vi "Obtain Broadcast Events.vi"(8 "error in (no error)":errorcluster, 10 "Create New?":bool) -> (0 "error out":errorcluster, 2 "Temperature-Module Broadcast Events":T1)   [LabVIEW 2021, in "Temperature-Module.lvlib"]
doc: "This VI Obtains/Creates the Broadcast events that will be used for other libraries to register to receive messages from the library that owns this VI.\n\n<b>NOTE</b>: The contents of this VI are automatically generated and modified by the <b>Tools > Delacor > User Event</b> utilities. Consider using those utilities instead of making your own modifications to this VI.\n_______\nCreated using Delacor User Event Scripter 1.0.0.6."
uses:
  Temperature-Module.lvlib
  Broadcast Events--cluster.ctl
  Status Updated Argument--cluster.ctl
  Send Temperature to HMI Argument--cluster.ctl
panel:
  # "NOTE: The contents of this VI are automatically generated and modified by the Tools > Delacor > User Event utilities. Consider using those utilities instead of making your own modifications to this VI."
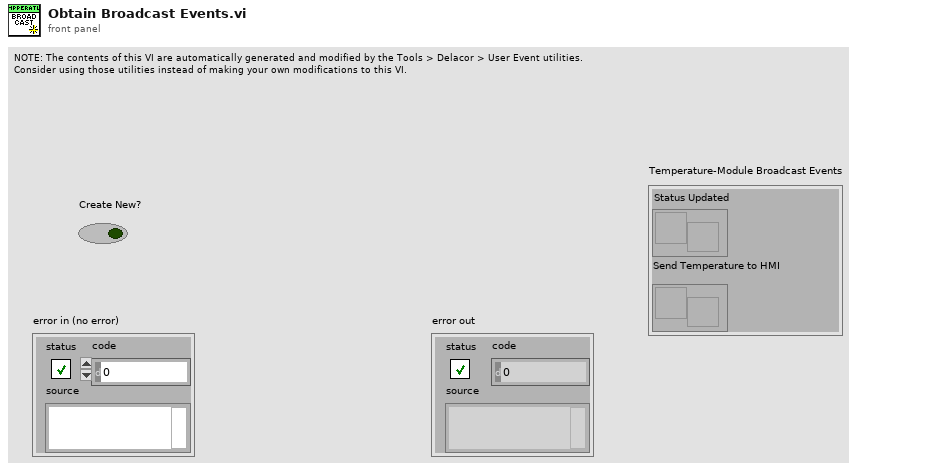
[diagram p1: front panel]
types:
  T1 = typedef "Temperature-Module.lvlib/Broadcast Events--cluster.ctl" = cluster{"Status Updated":refnum<user-event>, "Send Temperature to HMI":refnum<user-event>}
  T2 = typedef "Temperature-Module.lvlib/Send Temperature to HMI Argument--cluster.ctl" = cluster{"Temperature":dbl[]}
  T3 = typedef "Temperature-Module.lvlib/Status Updated Argument--cluster.ctl" = cluster{"Status":string}
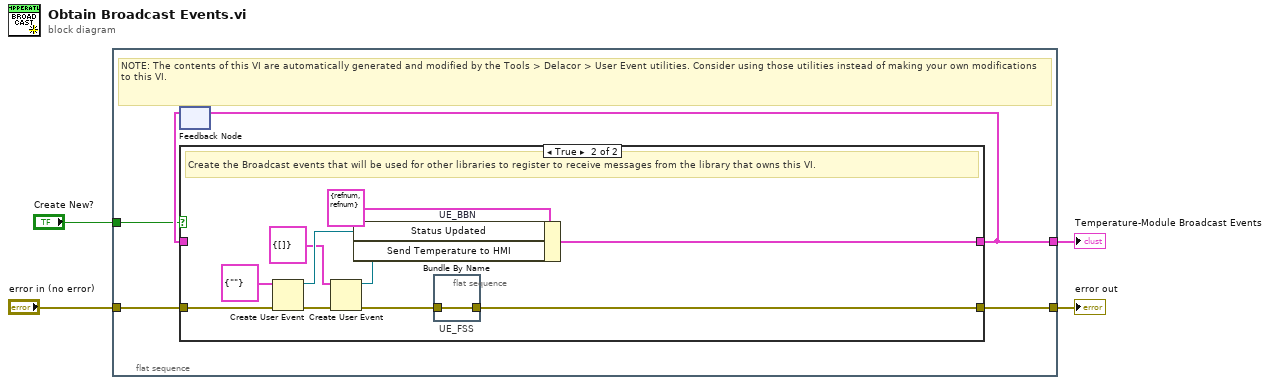
[diagram p0: block diagram]
diagram:
  n1 = flat-sequence {
    tunnel: [w9] -> w4
    tunnel: "error in (no error)" -> [w8]
    tunnel: [w6] -> w2
    tunnel: "Create New?" -> [w5]
    frame #0 {
      # "NOTE: The contents of this VI are automatically generated and modified by the Tools > Delacor > User Event utilities. Consider using those utilities instead of making your own modifications to this VI."
      n2 = feedback #1() -> (w7:T1)  [unwired: 1 in]
      n3 = case shown="True" w5 {
        tunnel: [w10 w15] -> w9
        tunnel: w8 -> [w10 w21]
        tunnel: [w11 w19] -> w6
        tunnel: w7 -> [w11 _]
        frame False {
          # "Obtain the Broadcast events that were created in a previous call to this VI."
        }
        frame True {
          # "Create the Broadcast events that will be used for other libraries to register to receive messages from the library that owns this VI."
          n4 = Create User Event(user event datatype=T3 {"Status"=""} ("Status Updated Argument"), error in=w21) -> (user event=w16:refnum<user-event>, error out=w18:errorcluster)
          n5 = Create User Event(user event datatype=T2 {"Temperature"=[]} ("Send Temperature to HMI Argument"), error in=w18) -> (user event=w13:refnum<user-event>, error out=w14:errorcluster)
          n6 = Bundle By Name "UE_BBN"(cluster=T1 {"Status Updated"=refnum, "Send Temperature to HMI"=refnum} ("output cluster"), "Status Updated"=w16, "Send Temperature to HMI"=w13) -> (w19:T1)
          n7 = flat-sequence "UE_FSS" {
            tunnel: w14 -> [w22]
            tunnel: [w22] -> w15
            frame #0 {
            }
          }
        }
      }
      n8 = feedback-in #1(w6) -> ()
    }
  }
  "Temperature-Module Broadcast Events" <- w2
  "error out" <- w4
